vi "Search for Error File.vi"(8 "error in":errorcluster, 11 "File Patterns":string[](array[string])) -> (0 "error out":errorcluster, 3 "Error Files Paths":path[](array[path]))   [LabVIEW 2021]
doc: "Searches for all files that match given <b>File Patterns</b> input defaultly <b>(*errors.xml)</b> in application directory, its subfolders, current VI path and returns an array of <b>File Path</b> if found some. If no file is found, <b>error code 500 000 </b> is generated."
uses:
  c70a6b7f-f53f-4f2c-ad2b-d58987f3c762.vi
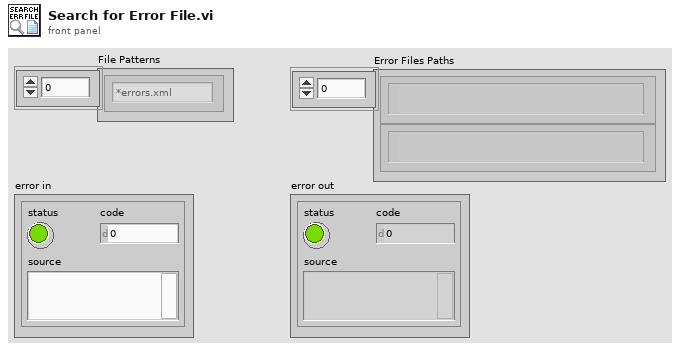
[diagram p1: front panel]
types:
  T1 = enum16{"open", "replace", "create", "open or create", "replace or create", "replace or create with confirmation"}
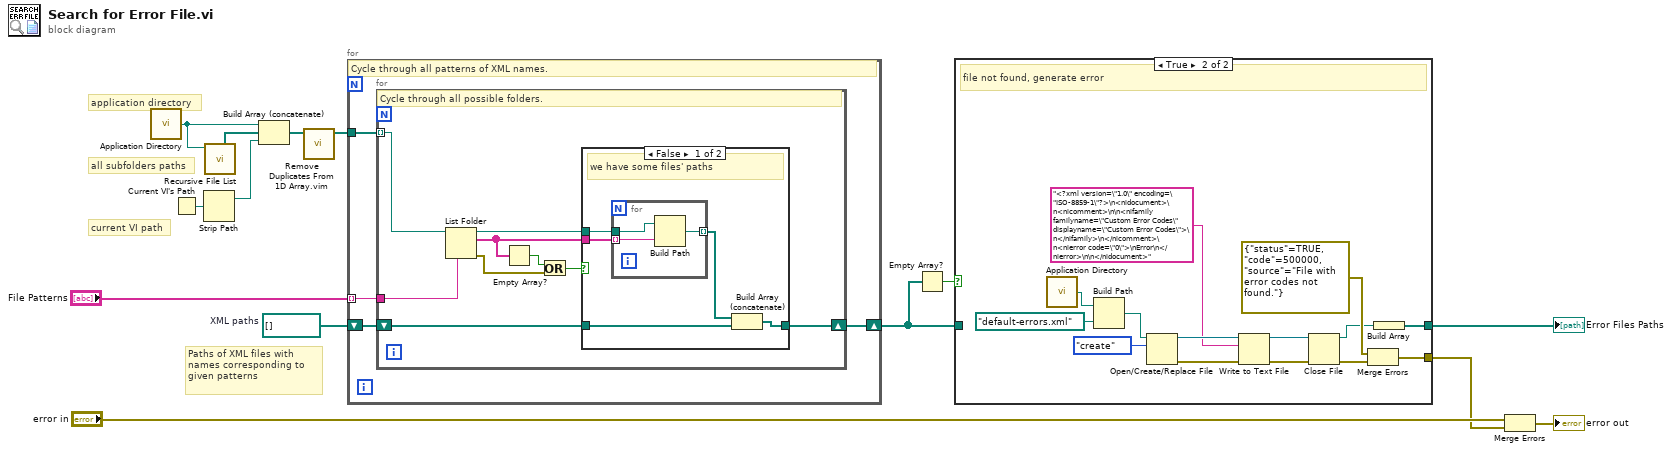
[diagram p0: block diagram]
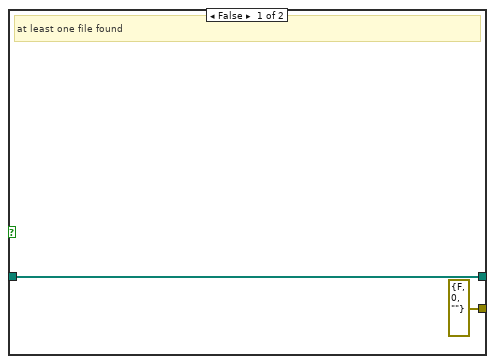
[diagram p2: hidden frame]
diagram:
  w9 = path[] []  # XML paths
  # "Paths of XML files with names corresponding to given patterns"
  # "application directory"
  # "current VI path"
  # "all subfolders paths"
  n1 = call <vilib>:"Application Directory.vi"() -> ("Application Directory"=w13:path)
  n2 = Current VI's Path() -> (path=w14:path)
  n3 = Strip Path(path=w14) -> (stripped path=w11:path)  [unwired: 1 out]
  n4 = call <vilib>:"Recursive File List.vi"("Folder Path"=w13) -> ("All Folders"=w12:path[])  [unwired: 6 in, 4 out]
  n5 = Build Array (concatenate)(w13, w12, w11) -> (w2:path[])
  n6 = call "Remove Duplicates From 1D Array.vim"("array"=w2) -> ("array with duplicates removed"=w1:path[])  [unwired: 10 in]
  n7 = for {
    tunnel: w1 -> [w18]
    tunnel: "File Patterns" -> [w17] mode=indexing
    shift-right: [w15] -> w6
    shift-left: w9 -> [w16]
    # "Cycle through all patterns of XML names."
    n8 = for {
      tunnel: w18 -> [w22] mode=indexing
      tunnel: w17 -> [w21]
      shift-right: [w19] -> w15
      shift-left: w16 -> [w20]
      # "Cycle through all possible folders."
      n9 = List Folder(path=w22, pattern=w21) -> (path out=w27:path, filenames=w26:string[], error out=w24:errorcluster)  [unwired: 2 in, 1 out]
      n10 = Empty Array?(array=w26) -> (empty?=w25:bool)
      n11 = Or(x=w25, y=w24) -> (x .or. y?=w23:bool)
      n12 = case shown="False" w23 {
        tunnel: w27 -> [w32 _]
        tunnel: w26 -> [w31 _]
        tunnel: w20 -> [w30 w36]
        tunnel: [w28 w36] -> w19
        frame False {
          # "we have some files' paths"
          n13 = for {
            tunnel: w32 -> [w35]
            tunnel: w31 -> [w34] mode=indexing
            tunnel: [w33] -> w29 mode=indexing
            n14 = Build Path(base path=w35, name or relative path=w34) -> (appended path=w33:path)
          }
          n15 = Build Array (concatenate)(w29, w30) -> (w28:path[])
        }
        frame True {
          # "no file OR error"
        }
      }
    }
  }
  n16 = Empty Array?(array=w6) -> (empty?=w8:bool)
  n17 = case shown="True" w8 {
    tunnel: [errorcluster {"status"=FALSE, "code"=0, "source"=""} ("error IO") w42] -> w3
    tunnel: [w38 w39] -> w7
    tunnel: w6 -> [w38 _]
    frame False {
      # "at least one file found"
    }
    frame True {
      # "file not found, generate error"
      n18 = call <vilib>:"Application Directory.vi"() -> ("Application Directory"=w49:path)
      n19 = Build Path(base path=w49, name or relative path=path "default-errors.xml") -> (appended path=w47:path)
      n20 = Open/Create/Replace File(file path (use dialog)=w47, operation (0:open)=T1."create") -> (refnum out=w51:refnum<file>, error out=w50:errorcluster)  [unwired: 4 in, 1 out]
      n21 = Write to Text File(file (use dialog)=w51, text="<?xml version=\"1.0\" encoding=\"ISO-8859-1\"?>\n<nidocument>\n<nicomment>\n\n<nifamily familyname=\"Custom Error Codes\" displayname=\"Custom Error Codes\">\n</nifamily>\n</nicomment>\n<nierror code=\"0\">\nError\n</nierror>\n\n</nidocument>", error in=w50) -> (refnum out=w45:refnum<file>, error out=w46:errorcluster)  [unwired: 1 in, 1 out]
      n22 = Close File(refnum=w45, error in=w46) -> (path=w41:path, error out=w44:errorcluster)
      n23 = Merge Errors(errorcluster {"status"=TRUE, "code"=500000, "source"="File with error codes not found."} ("error out"), w44) -> (w42:errorcluster)
      n24 = Build Array(w41) -> (w39:path[])
    }
  }
  "Error Files Paths" <- w7
  n25 = Merge Errors("error in", w3) -> (→"error out":errorcluster)
